vi "iPSset.vi"(7 "Field Rate, T/min":dbl, 8 "error in (no error)":errorcluster, 9 "Target Field, T":dbl, 10 "iPSSetCtrl":T1, 11 "VISA resource name":refnum<visa-resource-name>) -> (0 "error out":errorcluster, 1 "read buffer":string, 2 "number":dbl, 3 "VISA resource name out":refnum<visa-resource-name>)   [LabVIEW 2017]
uses:
  controls/iPSsetCtrl.ctl
  <vilib>/regexp/Match Regular Expression.xnode
panel:
  out "call chain":string[](array[string])
  out "concatenated string 2":string
  out "concatenated string":string
  out "after match":string
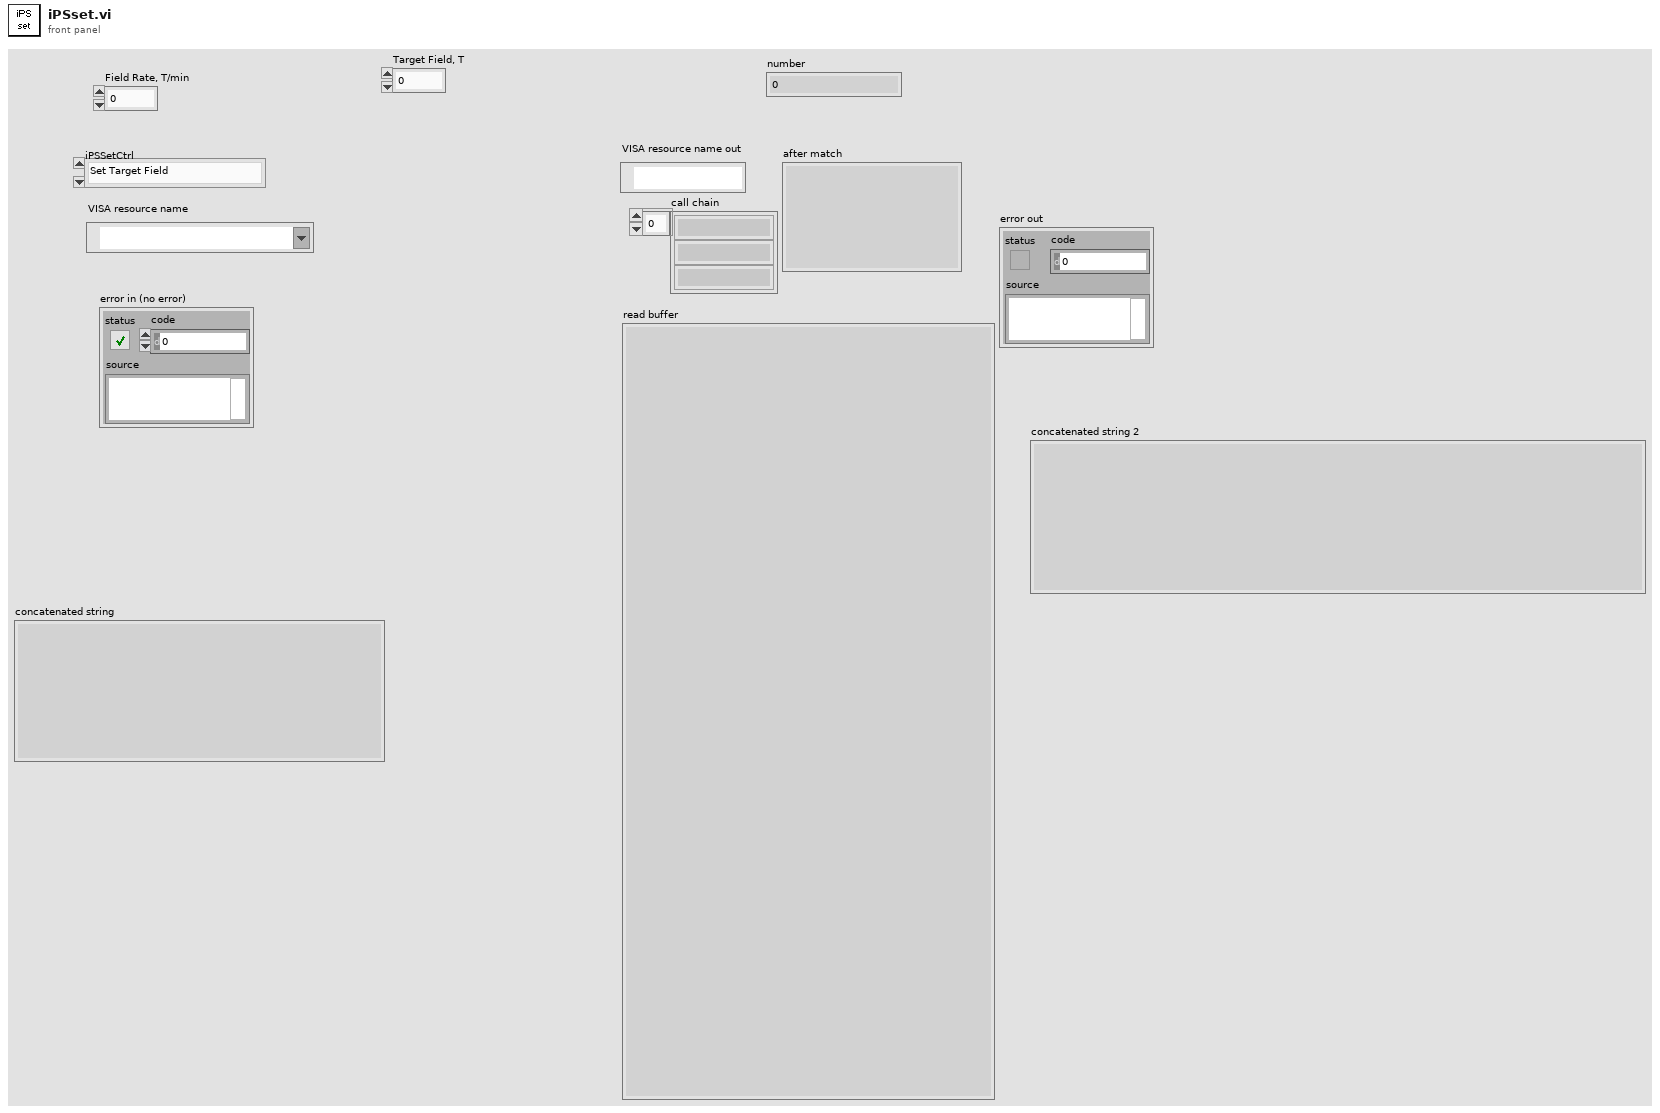
[diagram p1: front panel]
types:
  T1 = typedef "iPSsetCtrl.ctl" = enum16{"Set Target Field", "Set Target Field Rate", "Switch Heater ON", "Switch Heater OFF", "Go to Field", "Go to Zero", "Hold"}
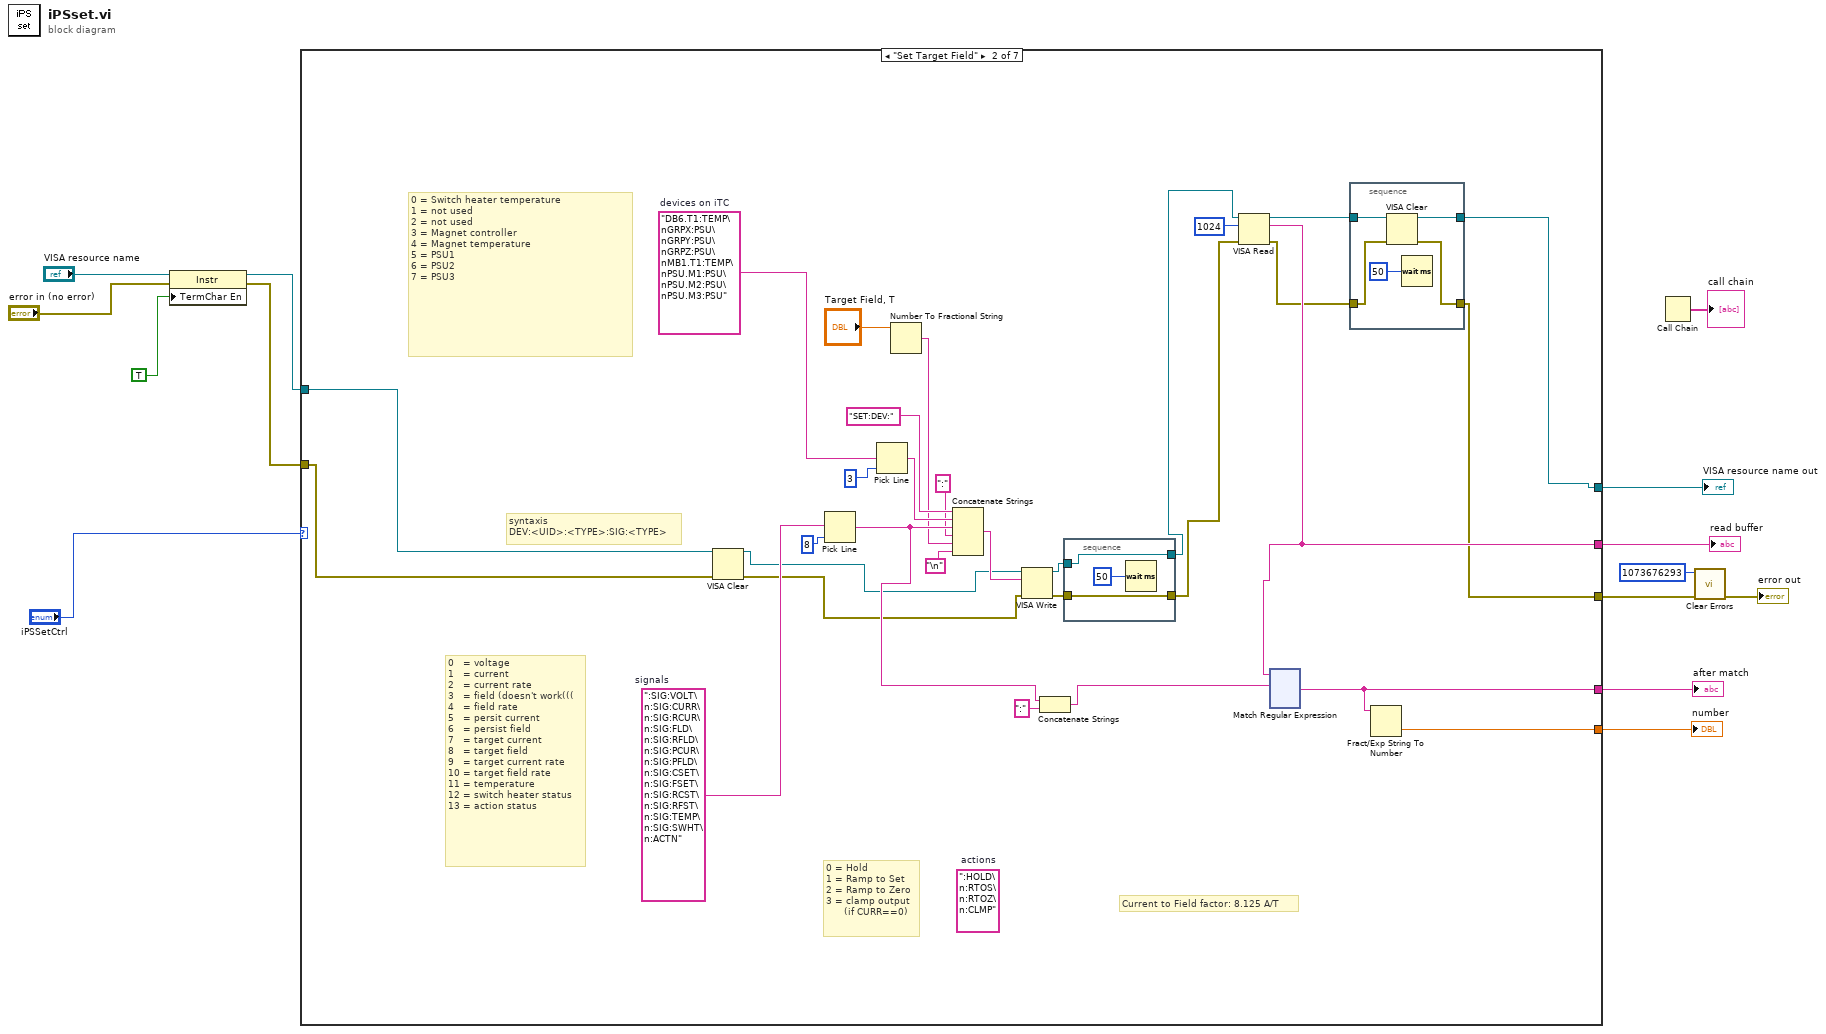
[diagram p0: block diagram]
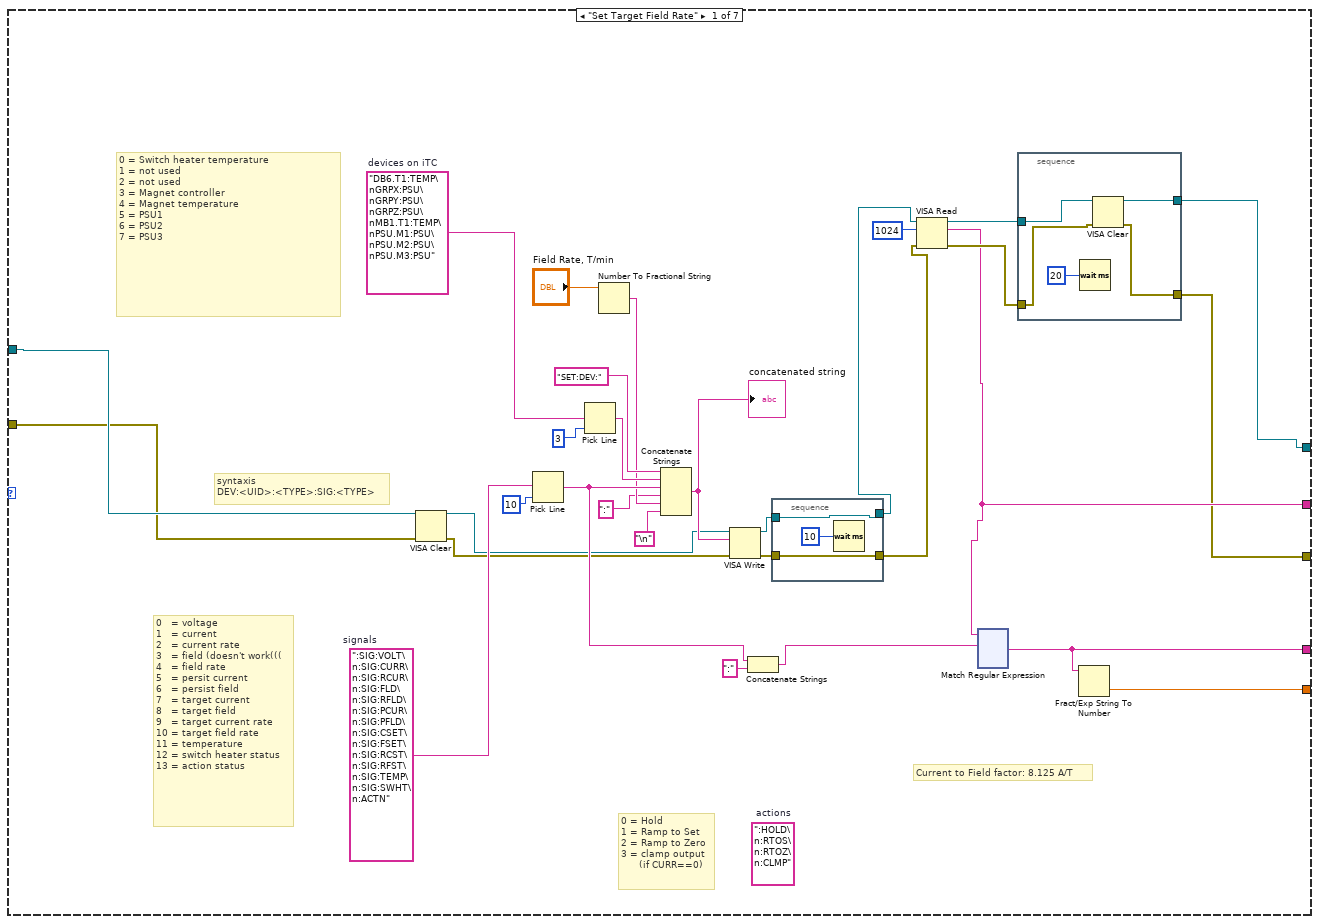
[diagram p2: hidden frame]
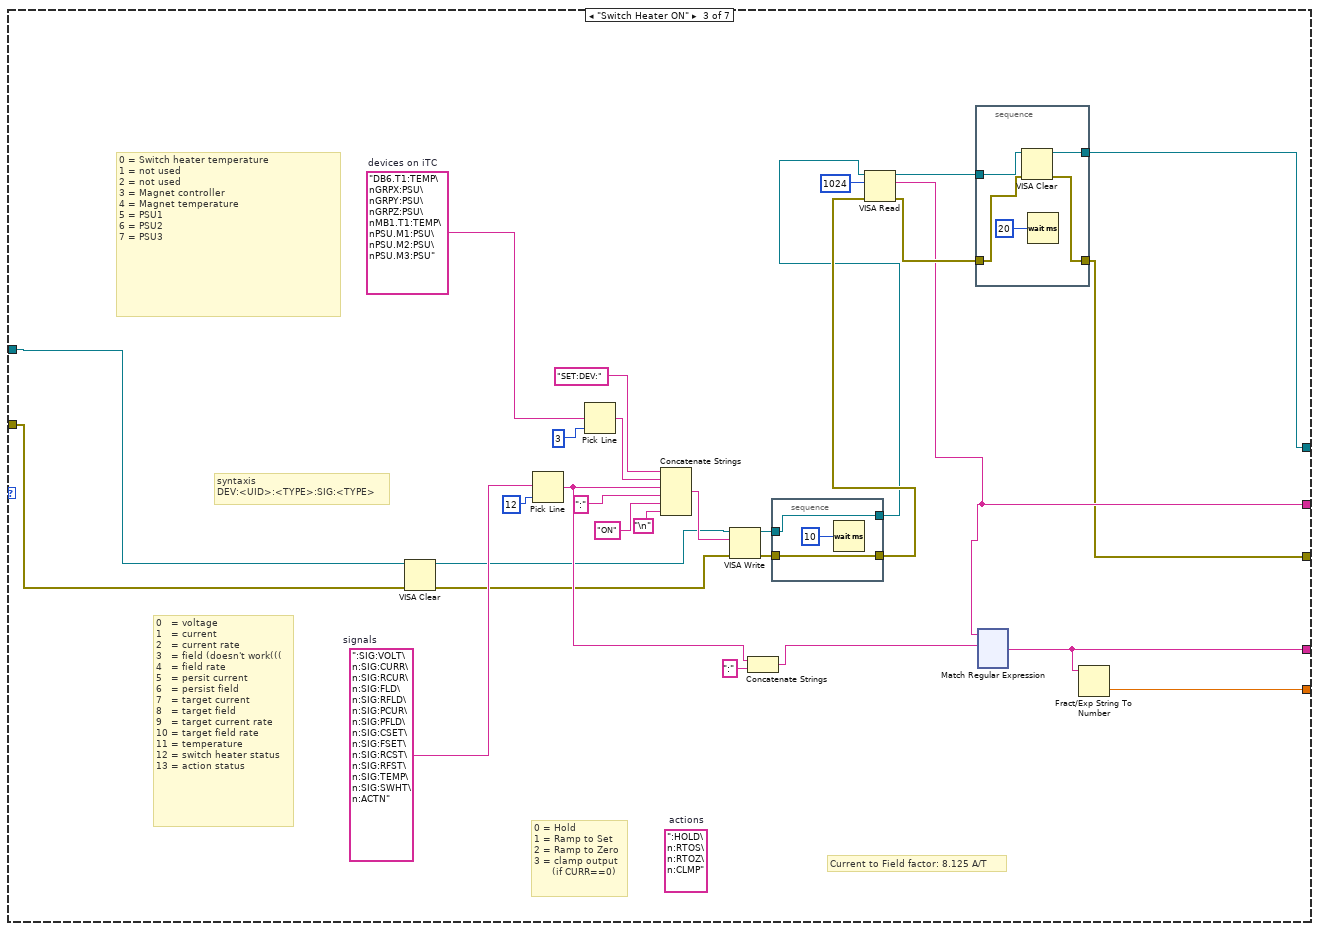
[diagram p3: hidden frame]
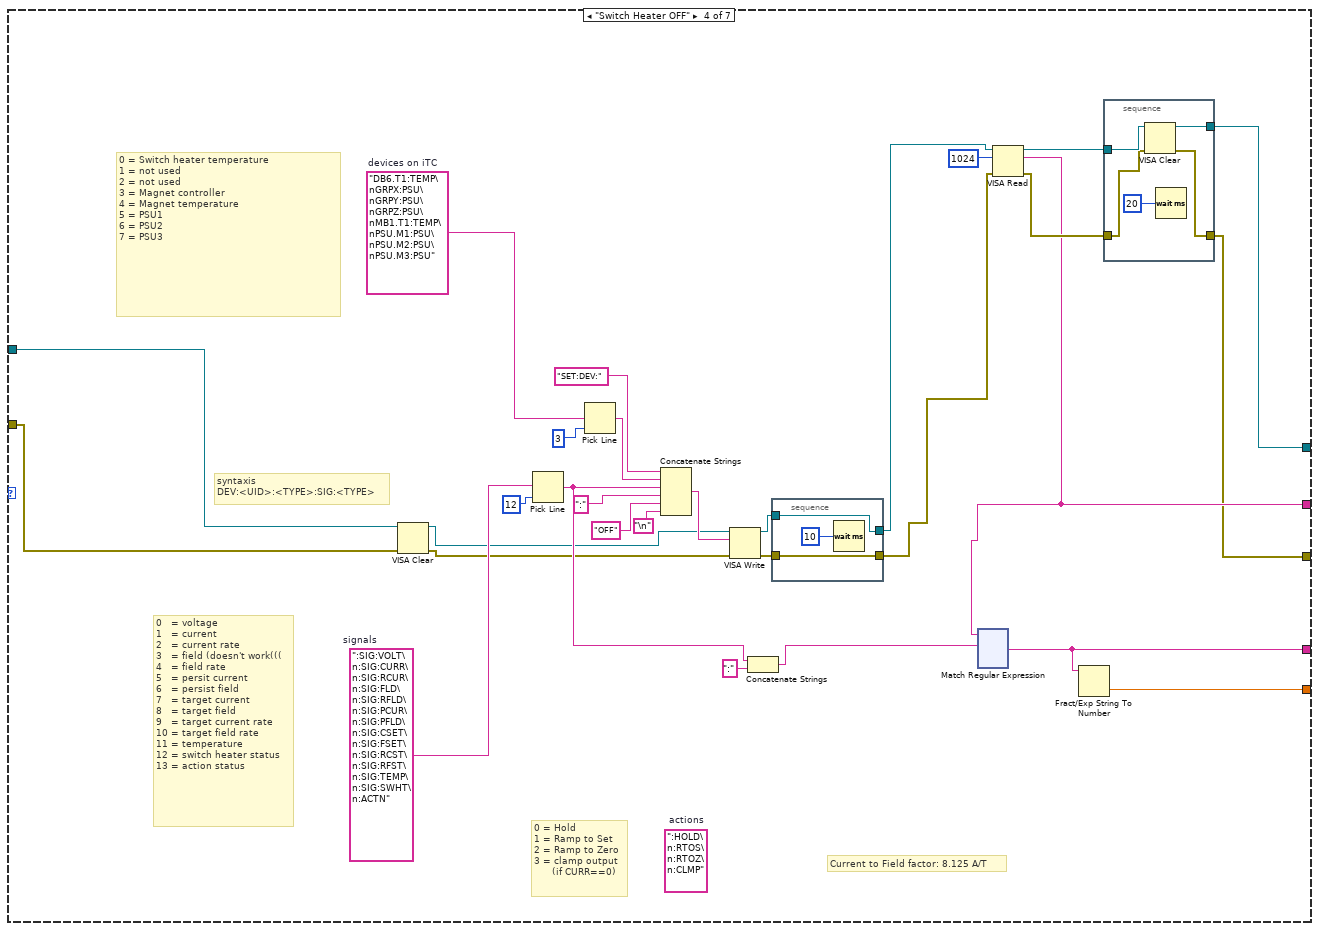
[diagram p4: hidden frame]
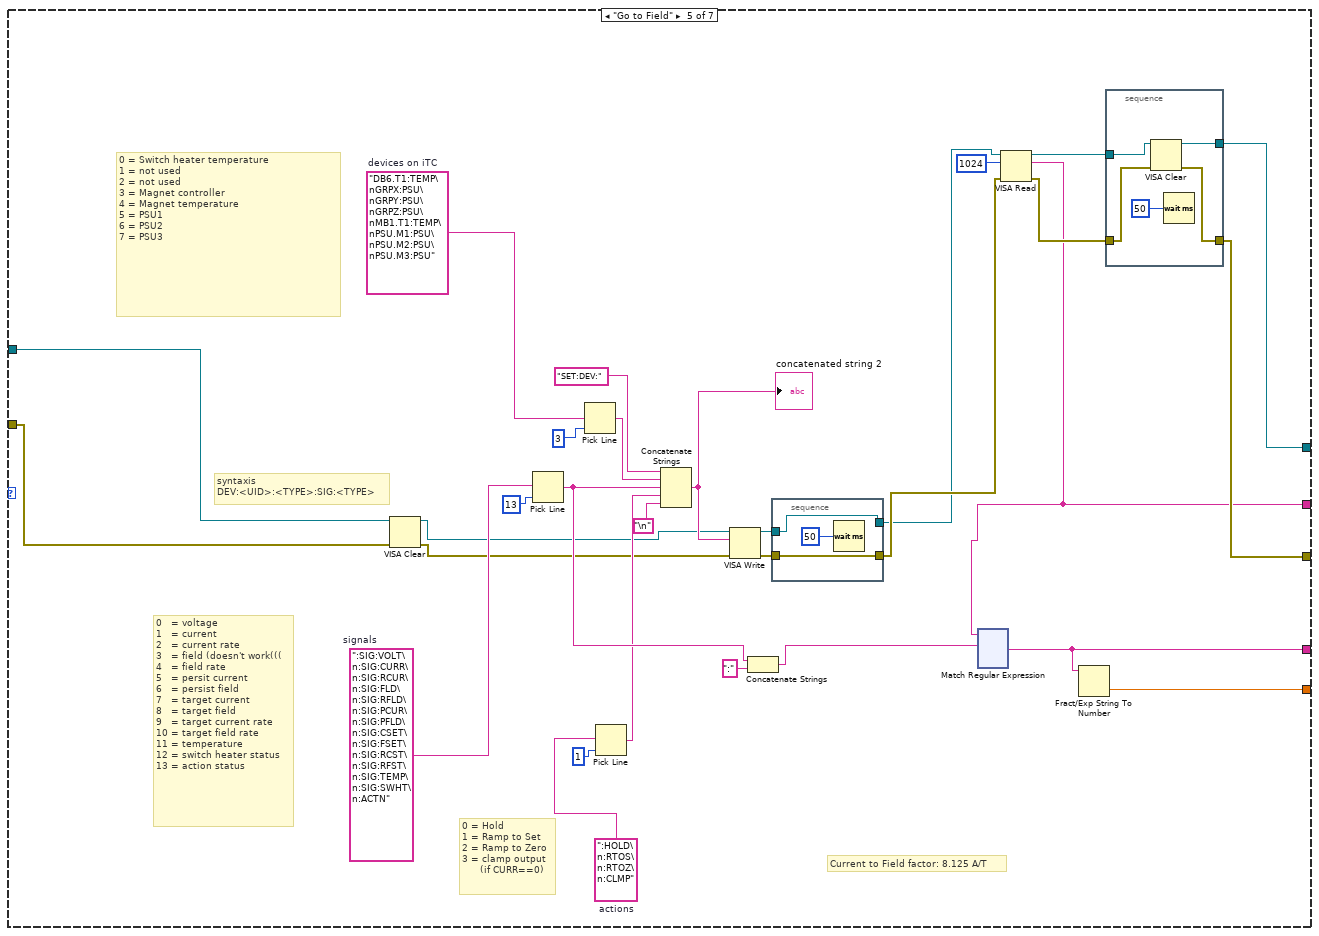
[diagram p5: hidden frame]
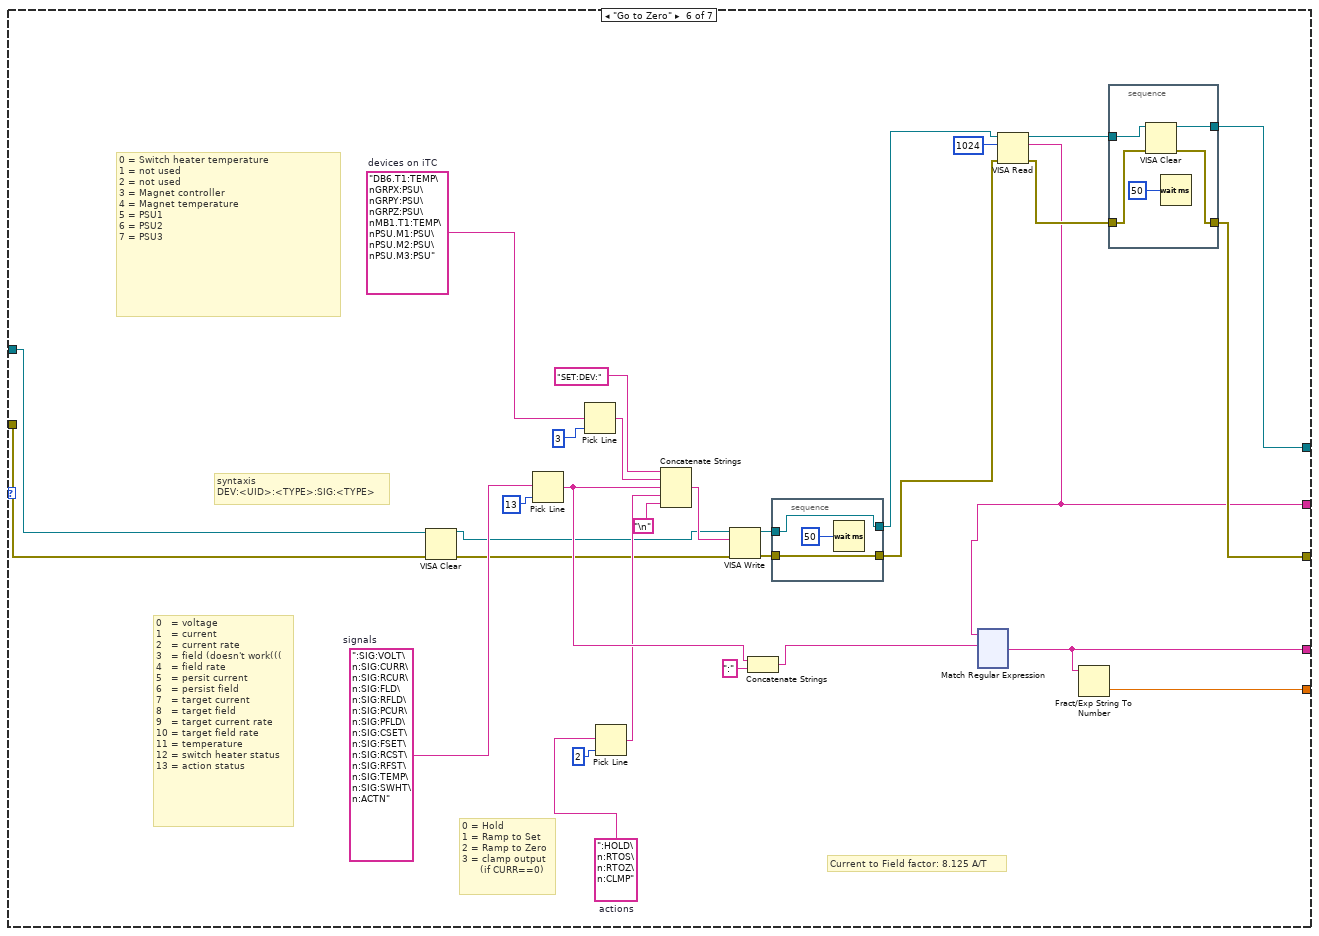
[diagram p6: hidden frame]
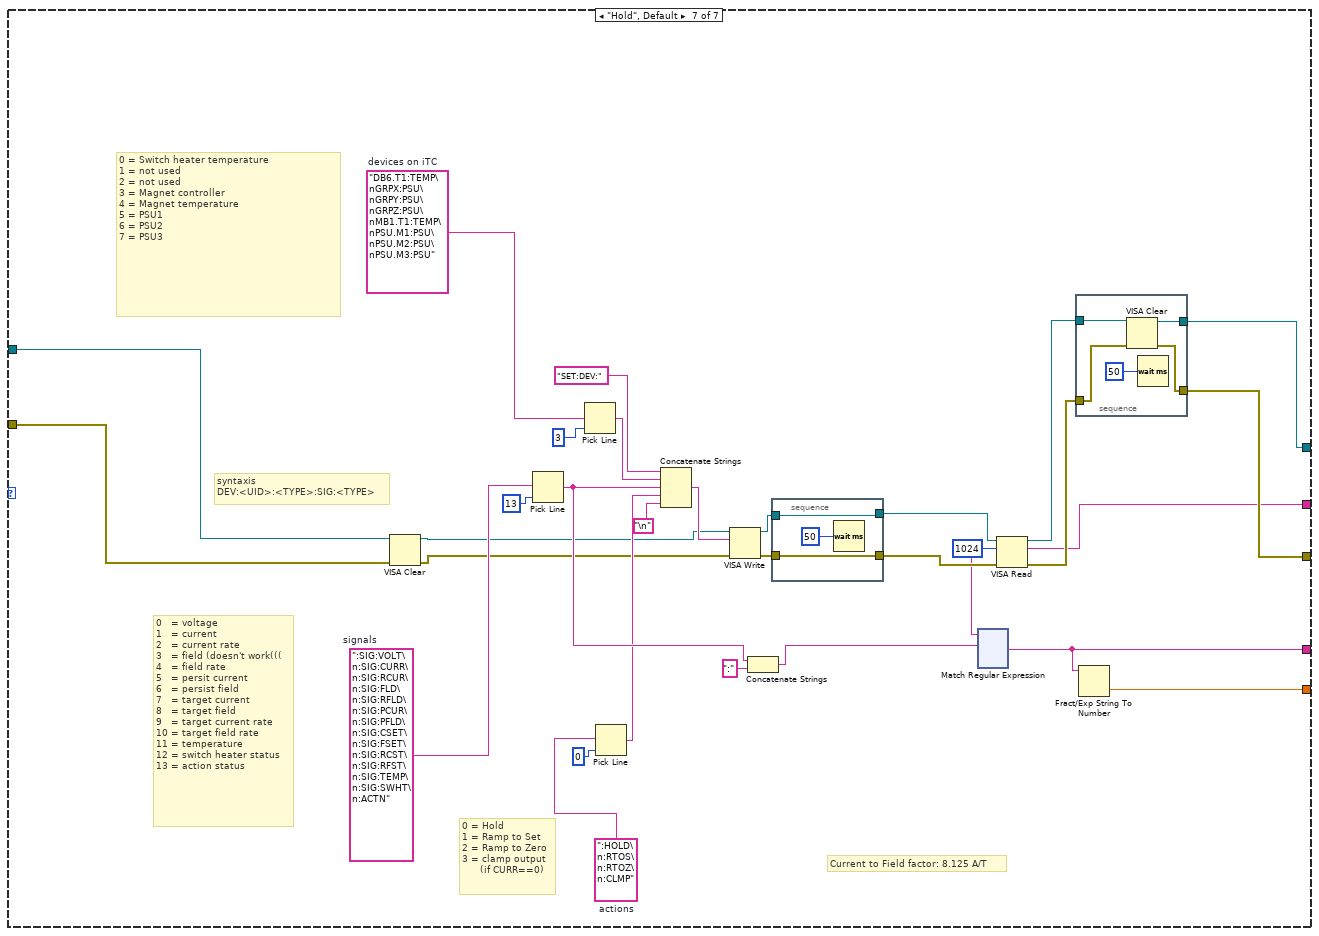
[diagram p7: hidden frame]
diagram:
  n1 = property class="Instr"(reference="VISA resource name", error in="error in (no error)", "TermChar En"=TRUE ("Message Based Settings:Termination Character Enable")) -> (reference out=w8:refnum<visa-resource-name>, error out=w7:errorcluster)
  n2 = case shown="\"Set Target Field\"" "iPSSetCtrl" {
    tunnel: [w23 w172 w321 w469 w619 w768 w916] -> w4
    tunnel: [w17 w166 w315 w463 w611 w761 w909] -> w14
    tunnel: [w24 w174 w322 w470 w618 w766 w915] -> w13
    tunnel: [w34 w183 w331 w479 w628 w777 w926] -> w12
    tunnel: [w33 w182 w330 w478 w627 w776 w925] -> w11
    tunnel: w7 -> [w21 w170 w319 w468 w616 w765 w914]
    tunnel: w8 -> [w22 w171 w320 w465 w614 w762 w911]
    frame "Set Target Field Rate" {
      (unwired) ":HOLD\n:RTOS\n:RTOZ\n:CLMP"  # actions
      w39 = ":SIG:VOLT\n:SIG:CURR\n:SIG:RCUR\n:SIG:FLD\n:SIG:RFLD\n:SIG:PCUR\n:SIG:PFLD\n:SIG:CSET\n:SIG:FSET\n:SIG:RCST\n:SIG:RFST\n:SIG:TEMP\n:SIG:SWHT\n:ACTN"  # signals
      w44 = "DB6.T1:TEMP\nGRPX:PSU\nGRPY:PSU\nGRPZ:PSU\nMB1.T1:TEMP\nPSU.M1:PSU\nPSU.M2:PSU\nPSU.M3:PSU"  # devices on iTC
      # "0 = Hold\n1 = Ramp to Set\n2 = Ramp to Zero\n3 = clamp output\n      (if CURR==0)"
      # "Current to Field factor: 8.125 A/T"
      # "0 = Switch heater temperature\n1 = not used\n2 = not used\n3 = Magnet controller \n4 = Magnet temperature\n5 = PSU1 \n6 = PSU2\n7 = PSU3"
      # "0   = voltage\n1   = current\n2   = current rate\n3   = field (doesn't work(((\n4   = field rate\n5   = persit current\n6   = persist field\n7   = target current\n8   = target field\n9   = target current rate\n10 = target field rate \n11 = temperature\n12 = switch heater status\n13 = action status"
      # "syntaxis\nDEV:<UID>:<TYPE>:SIG:<TYPE>"
      n3 = VISA Clear(VISA resource name=w22, error in (no error)=w21) -> (VISA resource name out=w19:refnum<visa-resource-name>, error out=w20:errorcluster)
      n4 = Pick Line(multi-line string=w39, line index=10) -> (output string=w37:string)  [unwired: 1 in]
      n5 = Pick Line(multi-line string=w44, line index=3) -> (output string=w41:string)  [unwired: 1 in]
      n6 = Number To Fractional String(number="Field Rate, T/min") -> (F-format string=w29:string)  [unwired: 3 in]
      n7 = Concatenate Strings("SET:DEV:" ("write buffer"), w41, w37, ":" ("string"), w29, "\n") -> (w35:string)
      "concatenated string" <- w35
      n8 = VISA Write(VISA resource name=w19, write buffer=w35, error in (no error)=w20) -> (VISA resource name out=w16:refnum<visa-resource-name>, error out=w43:errorcluster)  [unwired: 1 out]
      n9 = Concatenate Strings(w37, ":" ("string")) -> (w36:string)
      n10 = stacked-sequence {
        tunnel: w43 -> [w163]
        tunnel: [w163] -> w25
        tunnel: w16 -> [w161]
        tunnel: [w161] -> w15
        frame #0 {
          n11 = Wait (ms)(milliseconds to wait=u32 10) -> ()  [unwired: 1 out]
        }
      }
      n12 = VISA Read(VISA resource name=w15, byte count=u32 1024, error in (no error)=w25) -> (VISA resource name out=w18:refnum<visa-resource-name>, read buffer=w24:string, error out=w27:errorcluster)  [unwired: 1 out]
      n13 = xnode "Match Regular Expression"("input string"=w24, "regular expression"=w36) -> ("after match"=w34:string)  [unwired: 4 in, 4 out]
      n14 = stacked-sequence {
        tunnel: [w46] -> w23
        tunnel: w27 -> [w45]
        tunnel: w18 -> [w48]
        tunnel: [w47] -> w17
        frame #0 {
          n15 = Wait (ms)(milliseconds to wait=u32 20) -> ()  [unwired: 1 out]
          n16 = VISA Clear(VISA resource name=w48, error in (no error)=w45) -> (VISA resource name out=w47:refnum<visa-resource-name>, error out=w46:errorcluster)
        }
      }
      n17 = Fract/Exp String To Number(string=w34) -> (number=w33:dbl)  [unwired: 3 in, 1 out]
    }
    frame "Set Target Field" {
      (unwired) ":HOLD\n:RTOS\n:RTOZ\n:CLMP"  # actions
      w188 = ":SIG:VOLT\n:SIG:CURR\n:SIG:RCUR\n:SIG:FLD\n:SIG:RFLD\n:SIG:PCUR\n:SIG:PFLD\n:SIG:CSET\n:SIG:FSET\n:SIG:RCST\n:SIG:RFST\n:SIG:TEMP\n:SIG:SWHT\n:ACTN"  # signals
      w193 = "DB6.T1:TEMP\nGRPX:PSU\nGRPY:PSU\nGRPZ:PSU\nMB1.T1:TEMP\nPSU.M1:PSU\nPSU.M2:PSU\nPSU.M3:PSU"  # devices on iTC
      # "0 = Hold\n1 = Ramp to Set\n2 = Ramp to Zero\n3 = clamp output\n      (if CURR==0)"
      # "Current to Field factor: 8.125 A/T"
      # "0 = Switch heater temperature\n1 = not used\n2 = not used\n3 = Magnet controller \n4 = Magnet temperature\n5 = PSU1 \n6 = PSU2\n7 = PSU3"
      # "0   = voltage\n1   = current\n2   = current rate\n3   = field (doesn't work(((\n4   = field rate\n5   = persit current\n6   = persist field\n7   = target current\n8   = target field\n9   = target current rate\n10 = target field rate \n11 = temperature\n12 = switch heater status\n13 = action status"
      # "syntaxis\nDEV:<UID>:<TYPE>:SIG:<TYPE>"
      n18 = VISA Clear(VISA resource name=w171, error in (no error)=w170) -> (VISA resource name out=w168:refnum<visa-resource-name>, error out=w169:errorcluster)
      n19 = Pick Line(multi-line string=w188, line index=8) -> (output string=w186:string)  [unwired: 1 in]
      n20 = Pick Line(multi-line string=w193, line index=3) -> (output string=w190:string)  [unwired: 1 in]
      n21 = Number To Fractional String(number="Target Field, T") -> (F-format string=w178:string)  [unwired: 3 in]
      n22 = Concatenate Strings("SET:DEV:" ("write buffer"), w190, w186, ":" ("string"), w178, "\n") -> (w184:string)
      n23 = VISA Write(VISA resource name=w168, write buffer=w184, error in (no error)=w169) -> (VISA resource name out=w165:refnum<visa-resource-name>, error out=w192:errorcluster)  [unwired: 1 out]
      n24 = Concatenate Strings(w186, ":" ("string")) -> (w185:string)
      n25 = stacked-sequence {
        tunnel: w192 -> [w312]
        tunnel: [w312] -> w175
        tunnel: w165 -> [w310]
        tunnel: [w310] -> w164
        frame #0 {
          n26 = Wait (ms)(milliseconds to wait=u32 50) -> ()  [unwired: 1 out]
        }
      }
      n27 = VISA Read(VISA resource name=w164, byte count=u32 1024, error in (no error)=w175) -> (VISA resource name out=w167:refnum<visa-resource-name>, read buffer=w174:string, error out=w173:errorcluster)  [unwired: 1 out]
      n28 = xnode "Match Regular Expression"("input string"=w174, "regular expression"=w185) -> ("after match"=w183:string)  [unwired: 4 in, 4 out]
      n29 = stacked-sequence {
        tunnel: w173 -> [w196]
        tunnel: [w195] -> w172
        tunnel: w167 -> [w197]
        tunnel: [w194] -> w166
        frame #0 {
          n30 = VISA Clear(VISA resource name=w197, error in (no error)=w196) -> (VISA resource name out=w194:refnum<visa-resource-name>, error out=w195:errorcluster)
          n31 = Wait (ms)(milliseconds to wait=u32 50) -> ()  [unwired: 1 out]
        }
      }
      n32 = Fract/Exp String To Number(string=w183) -> (number=w182:dbl)  [unwired: 3 in, 1 out]
    }
    frame "Switch Heater ON" {
      (unwired) ":HOLD\n:RTOS\n:RTOZ\n:CLMP"  # actions
      w336 = ":SIG:VOLT\n:SIG:CURR\n:SIG:RCUR\n:SIG:FLD\n:SIG:RFLD\n:SIG:PCUR\n:SIG:PFLD\n:SIG:CSET\n:SIG:FSET\n:SIG:RCST\n:SIG:RFST\n:SIG:TEMP\n:SIG:SWHT\n:ACTN"  # signals
      w341 = "DB6.T1:TEMP\nGRPX:PSU\nGRPY:PSU\nGRPZ:PSU\nMB1.T1:TEMP\nPSU.M1:PSU\nPSU.M2:PSU\nPSU.M3:PSU"  # devices on iTC
      # "0 = Hold\n1 = Ramp to Set\n2 = Ramp to Zero\n3 = clamp output\n      (if CURR==0)"
      # "Current to Field factor: 8.125 A/T"
      # "0 = Switch heater temperature\n1 = not used\n2 = not used\n3 = Magnet controller \n4 = Magnet temperature\n5 = PSU1 \n6 = PSU2\n7 = PSU3"
      # "0   = voltage\n1   = current\n2   = current rate\n3   = field (doesn't work(((\n4   = field rate\n5   = persit current\n6   = persist field\n7   = target current\n8   = target field\n9   = target current rate\n10 = target field rate \n11 = temperature\n12 = switch heater status\n13 = action status"
      # "syntaxis\nDEV:<UID>:<TYPE>:SIG:<TYPE>"
      n33 = VISA Clear(VISA resource name=w320, error in (no error)=w319) -> (VISA resource name out=w317:refnum<visa-resource-name>, error out=w318:errorcluster)
      n34 = Pick Line(multi-line string=w336, line index=12) -> (output string=w334:string)  [unwired: 1 in]
      n35 = Pick Line(multi-line string=w341, line index=3) -> (output string=w338:string)  [unwired: 1 in]
      n36 = Concatenate Strings("SET:DEV:" ("write buffer"), w338, w334, ":" ("string"), "ON" ("string"), "\n") -> (w332:string)
      n37 = VISA Write(VISA resource name=w317, write buffer=w332, error in (no error)=w318) -> (VISA resource name out=w313:refnum<visa-resource-name>, error out=w340:errorcluster)  [unwired: 1 out]
      n38 = Concatenate Strings(w334, ":" ("string")) -> (w333:string)
      n39 = stacked-sequence {
        tunnel: w340 -> [w460]
        tunnel: [w460] -> w323
        tunnel: [w458] -> w314
        tunnel: w313 -> [w458]
        frame #0 {
          n40 = Wait (ms)(milliseconds to wait=u32 10) -> ()  [unwired: 1 out]
        }
      }
      n41 = VISA Read(VISA resource name=w314, byte count=u32 1024, error in (no error)=w323) -> (VISA resource name out=w316:refnum<visa-resource-name>, read buffer=w322:string, error out=w324:errorcluster)  [unwired: 1 out]
      n42 = stacked-sequence {
        tunnel: w324 -> [w342]
        tunnel: [w343] -> w321
        tunnel: w316 -> [w345]
        tunnel: [w344] -> w315
        frame #0 {
          n43 = VISA Clear(VISA resource name=w345, error in (no error)=w342) -> (VISA resource name out=w344:refnum<visa-resource-name>, error out=w343:errorcluster)
          n44 = Wait (ms)(milliseconds to wait=u32 20) -> ()  [unwired: 1 out]
        }
      }
      n45 = xnode "Match Regular Expression"("input string"=w322, "regular expression"=w333) -> ("after match"=w331:string)  [unwired: 4 in, 4 out]
      n46 = Fract/Exp String To Number(string=w331) -> (number=w330:dbl)  [unwired: 3 in, 1 out]
    }
    frame "Switch Heater OFF" {
      (unwired) ":HOLD\n:RTOS\n:RTOZ\n:CLMP"  # actions
      w484 = ":SIG:VOLT\n:SIG:CURR\n:SIG:RCUR\n:SIG:FLD\n:SIG:RFLD\n:SIG:PCUR\n:SIG:PFLD\n:SIG:CSET\n:SIG:FSET\n:SIG:RCST\n:SIG:RFST\n:SIG:TEMP\n:SIG:SWHT\n:ACTN"  # signals
      w489 = "DB6.T1:TEMP\nGRPX:PSU\nGRPY:PSU\nGRPZ:PSU\nMB1.T1:TEMP\nPSU.M1:PSU\nPSU.M2:PSU\nPSU.M3:PSU"  # devices on iTC
      # "0 = Hold\n1 = Ramp to Set\n2 = Ramp to Zero\n3 = clamp output\n      (if CURR==0)"
      # "Current to Field factor: 8.125 A/T"
      # "0 = Switch heater temperature\n1 = not used\n2 = not used\n3 = Magnet controller \n4 = Magnet temperature\n5 = PSU1 \n6 = PSU2\n7 = PSU3"
      # "0   = voltage\n1   = current\n2   = current rate\n3   = field (doesn't work(((\n4   = field rate\n5   = persit current\n6   = persist field\n7   = target current\n8   = target field\n9   = target current rate\n10 = target field rate \n11 = temperature\n12 = switch heater status\n13 = action status"
      # "syntaxis\nDEV:<UID>:<TYPE>:SIG:<TYPE>"
      n47 = VISA Clear(VISA resource name=w465, error in (no error)=w468) -> (VISA resource name out=w466:refnum<visa-resource-name>, error out=w467:errorcluster)
      n48 = Pick Line(multi-line string=w484, line index=12) -> (output string=w482:string)  [unwired: 1 in]
      n49 = Pick Line(multi-line string=w489, line index=3) -> (output string=w486:string)  [unwired: 1 in]
      n50 = Concatenate Strings("SET:DEV:" ("write buffer"), w486, w482, ":" ("string"), "OFF" ("string"), "\n") -> (w480:string)
      n51 = VISA Write(VISA resource name=w466, write buffer=w480, error in (no error)=w467) -> (VISA resource name out=w462:refnum<visa-resource-name>, error out=w488:errorcluster)  [unwired: 1 out]
      n52 = Concatenate Strings(w482, ":" ("string")) -> (w481:string)
      n53 = stacked-sequence {
        tunnel: w488 -> [w608]
        tunnel: [w608] -> w471
        tunnel: [w606] -> w461
        tunnel: w462 -> [w606]
        frame #0 {
          n54 = Wait (ms)(milliseconds to wait=u32 10) -> ()  [unwired: 1 out]
        }
      }
      n55 = VISA Read(VISA resource name=w461, byte count=u32 1024, error in (no error)=w471) -> (VISA resource name out=w464:refnum<visa-resource-name>, read buffer=w470:string, error out=w472:errorcluster)  [unwired: 1 out]
      n56 = xnode "Match Regular Expression"("input string"=w470, "regular expression"=w481) -> ("after match"=w479:string)  [unwired: 4 in, 4 out]
      n57 = Fract/Exp String To Number(string=w479) -> (number=w478:dbl)  [unwired: 3 in, 1 out]
      n58 = stacked-sequence {
        tunnel: w472 -> [w490]
        tunnel: [w491] -> w469
        tunnel: w464 -> [w493]
        tunnel: [w492] -> w463
        frame #0 {
          n59 = VISA Clear(VISA resource name=w493, error in (no error)=w490) -> (VISA resource name out=w492:refnum<visa-resource-name>, error out=w491:errorcluster)
          n60 = Wait (ms)(milliseconds to wait=u32 20) -> ()  [unwired: 1 out]
        }
      }
    }
    frame "Go to Field" {
      w623 = ":HOLD\n:RTOS\n:RTOZ\n:CLMP"  # actions
      w633 = ":SIG:VOLT\n:SIG:CURR\n:SIG:RCUR\n:SIG:FLD\n:SIG:RFLD\n:SIG:PCUR\n:SIG:PFLD\n:SIG:CSET\n:SIG:FSET\n:SIG:RCST\n:SIG:RFST\n:SIG:TEMP\n:SIG:SWHT\n:ACTN"  # signals
      w638 = "DB6.T1:TEMP\nGRPX:PSU\nGRPY:PSU\nGRPZ:PSU\nMB1.T1:TEMP\nPSU.M1:PSU\nPSU.M2:PSU\nPSU.M3:PSU"  # devices on iTC
      # "0 = Hold\n1 = Ramp to Set\n2 = Ramp to Zero\n3 = clamp output\n      (if CURR==0)"
      # "Current to Field factor: 8.125 A/T"
      # "0 = Switch heater temperature\n1 = not used\n2 = not used\n3 = Magnet controller \n4 = Magnet temperature\n5 = PSU1 \n6 = PSU2\n7 = PSU3"
      # "0   = voltage\n1   = current\n2   = current rate\n3   = field (doesn't work(((\n4   = field rate\n5   = persit current\n6   = persist field\n7   = target current\n8   = target field\n9   = target current rate\n10 = target field rate \n11 = temperature\n12 = switch heater status\n13 = action status"
      # "syntaxis\nDEV:<UID>:<TYPE>:SIG:<TYPE>"
      n61 = VISA Clear(VISA resource name=w614, error in (no error)=w616) -> (VISA resource name out=w613:refnum<visa-resource-name>, error out=w615:errorcluster)
      n62 = Pick Line(multi-line string=w633, line index=13) -> (output string=w631:string)  [unwired: 1 in]
      n63 = Pick Line(multi-line string=w638, line index=3) -> (output string=w635:string)  [unwired: 1 in]
      n64 = Pick Line(multi-line string=w623, line index=1) -> (output string=w622:string)  [unwired: 1 in]
      n65 = Concatenate Strings("SET:DEV:" ("write buffer"), w635, w631, w622, "\n") -> (w629:string)
      "concatenated string 2" <- w629
      n66 = VISA Write(VISA resource name=w613, write buffer=w629, error in (no error)=w615) -> (VISA resource name out=w610:refnum<visa-resource-name>, error out=w637:errorcluster)  [unwired: 1 out]
      n67 = Concatenate Strings(w631, ":" ("string")) -> (w630:string)
      n68 = stacked-sequence {
        tunnel: w637 -> [w757]
        tunnel: [w757] -> w617
        tunnel: w610 -> [w755]
        tunnel: [w755] -> w609
        frame #0 {
          n69 = Wait (ms)(milliseconds to wait=u32 50) -> ()  [unwired: 1 out]
        }
      }
      n70 = VISA Read(VISA resource name=w609, byte count=u32 1024, error in (no error)=w617) -> (VISA resource name out=w612:refnum<visa-resource-name>, read buffer=w618:string, error out=w620:errorcluster)  [unwired: 1 out]
      n71 = xnode "Match Regular Expression"("input string"=w618, "regular expression"=w630) -> ("after match"=w628:string)  [unwired: 4 in, 4 out]
      n72 = Fract/Exp String To Number(string=w628) -> (number=w627:dbl)  [unwired: 3 in, 1 out]
      n73 = stacked-sequence {
        tunnel: w620 -> [w639]
        tunnel: [w640] -> w619
        tunnel: w612 -> [w642]
        tunnel: [w641] -> w611
        frame #0 {
          n74 = VISA Clear(VISA resource name=w642, error in (no error)=w639) -> (VISA resource name out=w641:refnum<visa-resource-name>, error out=w640:errorcluster)
          n75 = Wait (ms)(milliseconds to wait=u32 50) -> ()  [unwired: 1 out]
        }
      }
    }
    frame "Go to Zero" {
      w772 = ":HOLD\n:RTOS\n:RTOZ\n:CLMP"  # actions
      w782 = ":SIG:VOLT\n:SIG:CURR\n:SIG:RCUR\n:SIG:FLD\n:SIG:RFLD\n:SIG:PCUR\n:SIG:PFLD\n:SIG:CSET\n:SIG:FSET\n:SIG:RCST\n:SIG:RFST\n:SIG:TEMP\n:SIG:SWHT\n:ACTN"  # signals
      w787 = "DB6.T1:TEMP\nGRPX:PSU\nGRPY:PSU\nGRPZ:PSU\nMB1.T1:TEMP\nPSU.M1:PSU\nPSU.M2:PSU\nPSU.M3:PSU"  # devices on iTC
      # "0 = Hold\n1 = Ramp to Set\n2 = Ramp to Zero\n3 = clamp output\n      (if CURR==0)"
      # "Current to Field factor: 8.125 A/T"
      # "0 = Switch heater temperature\n1 = not used\n2 = not used\n3 = Magnet controller \n4 = Magnet temperature\n5 = PSU1 \n6 = PSU2\n7 = PSU3"
      # "0   = voltage\n1   = current\n2   = current rate\n3   = field (doesn't work(((\n4   = field rate\n5   = persit current\n6   = persist field\n7   = target current\n8   = target field\n9   = target current rate\n10 = target field rate \n11 = temperature\n12 = switch heater status\n13 = action status"
      # "syntaxis\nDEV:<UID>:<TYPE>:SIG:<TYPE>"
      n76 = VISA Clear(VISA resource name=w762, error in (no error)=w765) -> (VISA resource name out=w763:refnum<visa-resource-name>, error out=w764:errorcluster)
      n77 = Pick Line(multi-line string=w782, line index=13) -> (output string=w780:string)  [unwired: 1 in]
      n78 = Pick Line(multi-line string=w787, line index=3) -> (output string=w784:string)  [unwired: 1 in]
      n79 = Pick Line(multi-line string=w772, line index=2) -> (output string=w771:string)  [unwired: 1 in]
      n80 = Concatenate Strings("SET:DEV:" ("write buffer"), w784, w780, w771, "\n") -> (w778:string)
      n81 = VISA Write(VISA resource name=w763, write buffer=w778, error in (no error)=w764) -> (VISA resource name out=w759:refnum<visa-resource-name>, error out=w786:errorcluster)  [unwired: 1 out]
      n82 = Concatenate Strings(w780, ":" ("string")) -> (w779:string)
      n83 = stacked-sequence {
        tunnel: w786 -> [w906]
        tunnel: [w906] -> w767
        tunnel: w759 -> [w904]
        tunnel: [w904] -> w758
        frame #0 {
          n84 = Wait (ms)(milliseconds to wait=u32 50) -> ()  [unwired: 1 out]
        }
      }
      n85 = VISA Read(VISA resource name=w758, byte count=u32 1024, error in (no error)=w767) -> (VISA resource name out=w760:refnum<visa-resource-name>, read buffer=w766:string, error out=w769:errorcluster)  [unwired: 1 out]
      n86 = xnode "Match Regular Expression"("input string"=w766, "regular expression"=w779) -> ("after match"=w777:string)  [unwired: 4 in, 4 out]
      n87 = Fract/Exp String To Number(string=w777) -> (number=w776:dbl)  [unwired: 3 in, 1 out]
      n88 = stacked-sequence {
        tunnel: w769 -> [w789]
        tunnel: [w788] -> w768
        tunnel: [w791] -> w761
        tunnel: w760 -> [w790]
        frame #0 {
          n89 = VISA Clear(VISA resource name=w790, error in (no error)=w789) -> (VISA resource name out=w791:refnum<visa-resource-name>, error out=w788:errorcluster)
          n90 = Wait (ms)(milliseconds to wait=u32 50) -> ()  [unwired: 1 out]
        }
      }
    }
    frame "Hold", Default {
      w921 = ":HOLD\n:RTOS\n:RTOZ\n:CLMP"  # actions
      w931 = ":SIG:VOLT\n:SIG:CURR\n:SIG:RCUR\n:SIG:FLD\n:SIG:RFLD\n:SIG:PCUR\n:SIG:PFLD\n:SIG:CSET\n:SIG:FSET\n:SIG:RCST\n:SIG:RFST\n:SIG:TEMP\n:SIG:SWHT\n:ACTN"  # signals
      w936 = "DB6.T1:TEMP\nGRPX:PSU\nGRPY:PSU\nGRPZ:PSU\nMB1.T1:TEMP\nPSU.M1:PSU\nPSU.M2:PSU\nPSU.M3:PSU"  # devices on iTC
      # "0 = Hold\n1 = Ramp to Set\n2 = Ramp to Zero\n3 = clamp output\n      (if CURR==0)"
      # "Current to Field factor: 8.125 A/T"
      # "0 = Switch heater temperature\n1 = not used\n2 = not used\n3 = Magnet controller \n4 = Magnet temperature\n5 = PSU1 \n6 = PSU2\n7 = PSU3"
      # "0   = voltage\n1   = current\n2   = current rate\n3   = field (doesn't work(((\n4   = field rate\n5   = persit current\n6   = persist field\n7   = target current\n8   = target field\n9   = target current rate\n10 = target field rate \n11 = temperature\n12 = switch heater status\n13 = action status"
      # "syntaxis\nDEV:<UID>:<TYPE>:SIG:<TYPE>"
      n91 = VISA Clear(VISA resource name=w911, error in (no error)=w914) -> (VISA resource name out=w912:refnum<visa-resource-name>, error out=w913:errorcluster)
      n92 = Pick Line(multi-line string=w931, line index=13) -> (output string=w929:string)  [unwired: 1 in]
      n93 = Pick Line(multi-line string=w936, line index=3) -> (output string=w933:string)  [unwired: 1 in]
      n94 = Pick Line(multi-line string=w921, line index=0) -> (output string=w920:string)  [unwired: 1 in]
      n95 = Concatenate Strings("SET:DEV:" ("write buffer"), w933, w929, w920, "\n") -> (w927:string)
      n96 = VISA Write(VISA resource name=w912, write buffer=w927, error in (no error)=w913) -> (VISA resource name out=w908:refnum<visa-resource-name>, error out=w935:errorcluster)  [unwired: 1 out]
      n97 = Concatenate Strings(w929, ":" ("string")) -> (w928:string)
      n98 = stacked-sequence {
        tunnel: w935 -> [w1055]
        tunnel: [w1055] -> w918
        tunnel: [w1053] -> w907
        tunnel: w908 -> [w1053]
        frame #0 {
          n99 = Wait (ms)(milliseconds to wait=u32 50) -> ()  [unwired: 1 out]
        }
      }
      n100 = VISA Read(VISA resource name=w907, byte count=u32 1024, error in (no error)=w918) -> (VISA resource name out=w910:refnum<visa-resource-name>, read buffer=w915:string, error out=w917:errorcluster)  [unwired: 1 out]
      n101 = xnode "Match Regular Expression"("input string"=w915, "regular expression"=w928) -> ("after match"=w926:string)  [unwired: 4 in, 4 out]
      n102 = stacked-sequence {
        tunnel: [w938] -> w916
        tunnel: w917 -> [w939]
        tunnel: w910 -> [w940]
        tunnel: [w937] -> w909
        frame #0 {
          n103 = VISA Clear(VISA resource name=w940, error in (no error)=w939) -> (VISA resource name out=w937:refnum<visa-resource-name>, error out=w938:errorcluster)
          n104 = Wait (ms)(milliseconds to wait=u32 50) -> ()  [unwired: 1 out]
        }
      }
      n105 = Fract/Exp String To Number(string=w926) -> (number=w925:dbl)  [unwired: 3 in, 1 out]
    }
  }
  "read buffer" <- w13
  "VISA resource name out" <- w14
  "after match" <- w12
  "number" <- w11
  n106 = Call Chain() -> (call chain=→"call chain":string[])
  n107 = call <vilib>:"Clear Errors.vi"("error in (no error)"=w4, "specific error code to clear (0: all)"=1073676293) -> ("error out"=→"error out":errorcluster)  [unwired: 4 in, 1 out]
